vi "Pickup Floor.vi"(11 "Final Height":dbl format="%#_13g") -> ()   [LabVIEW 2014]
uses:
  Begin/Global Variables.vi
panel:
  in  "Slow":dbl=0.6
  in  "Fast":dbl=0.75
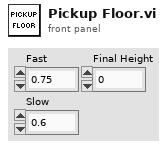
[diagram p1: front panel]
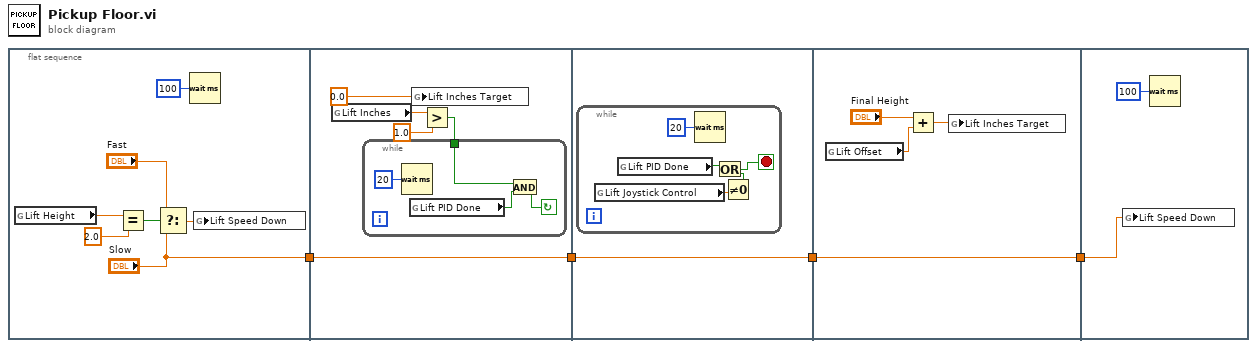
[diagram p0: block diagram]
diagram:
  n1 = flat-sequence {
    tunnel: ["Slow"] -> w1
    tunnel: [w12] -> w2
    tunnel: w1 -> [w12]
    tunnel: [w21] -> w3
    tunnel: w2 -> [w21]
    tunnel: [w27] -> w4
    tunnel: w3 -> [w27]
    tunnel: w4 -> [w31]
    frame #0 {
      n2 = global read "Global Variables.vi" "Lift Height"() -> (w10:dbl)
      n3 = Equal?(x=w10, y=2.0) -> (x = y?=w8:bool)
      n4 = Select(t="Fast", s=w8, f="Slow") -> (s? t:f=w7:dbl)
      n5 = Wait (ms)(milliseconds to wait=u32 100) -> ()  [unwired: 1 out]
      n6 = global write "Global Variables.vi" "Lift Speed Down"(w7) -> ()
    }
    frame #1 {
      n7 = global read "Global Variables.vi" "Lift Inches"() -> (w14:dbl)
      n8 = global write "Global Variables.vi" "Lift Inches Target"(0.0 ("x")) -> ()
      n9 = Greater?(x=w14, y=1.0) -> (0:w13:bool)
      n10 = while {
        tunnel: w13 -> [w17]
        stop <- w18 continue-if-true
        n11 = Wait (ms)(milliseconds to wait=u32 20) -> ()  [unwired: 1 out]
        n12 = global read "Global Variables.vi" "Lift PID Done"() -> (w19:bool)
        n13 = And(x=w17, y=w19) -> (x .and. y?=w18:bool)
      }
    }
    frame #2 {
      n14 = while {
        stop <- w22 stop-if-true
        n15 = global read "Global Variables.vi" "Lift Joystick Control"() -> (w25:dbl)
        n16 = global read "Global Variables.vi" "Lift PID Done"() -> (w23:bool)
        n17 = Wait (ms)(milliseconds to wait=u32 20) -> ()  [unwired: 1 out]
        n18 = Not Equal To 0?(x=w25) -> (x != 0?=w24:bool)
        n19 = Or(x=w23, y=w24) -> (x .or. y?=w22:bool)
      }
    }
    frame #3 {
      n20 = global read "Global Variables.vi" "Lift Offset"() -> (w29:dbl)
      n21 = Add(x="Final Height", y=w29) -> (x+y=w30:dbl)
      n22 = global write "Global Variables.vi" "Lift Inches Target"(w30) -> ()
    }
    frame #4 {
      n23 = global write "Global Variables.vi" "Lift Speed Down"(w31) -> ()
      n24 = Wait (ms)(milliseconds to wait=u32 100) -> ()  [unwired: 1 out]
    }
  }
